vi "Callback Confirm Start.vi"(4 "Variant":variant, 6 "Control Ref":refnum<k7>, 7 "Event Common Data":T1) -> ()   [LabVIEW 2014]
uses:
  support/Message Queue/All Message Queues.ctl
  support/Message Queue/Message Cluster.ctl
  support/Message Queue/Enqueue Message (Single).vi
  support/Message Queue/Message Queue.lvlib
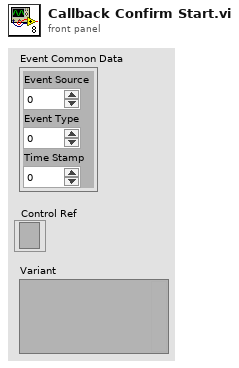
[diagram p1: front panel]
types:
  T1 = cluster{"Event Source":i32, "Event Type":u32, "Time Stamp":u32}
  T2 = typedef "Message Queue.lvlib/All Message Queues.ctl" = cluster{"UI":refnum<queue>, "Engine":refnum<queue>, "Laser":refnum<queue>, "Keyence":refnum<queue>, "Data Processor":refnum<queue>, "Timers":refnum<queue>, "Timer mérés":refnum<queue>, "Timer laser":refnum<queue>, "DAQ":refnum<queue>, "NI Digital":refnum<queue>, "DI data":refnum<queue>, "DO data":refnum<queue>, "Data Processor data":refnum<queue>, "Keyence Data":refnum<queue>, "Ring":refnum<queue>, "NI Analog":refnum<queue>, "AI data":refnum<queue>, "AO data":refnum<queue>, "Analog UI Data":refnum<queue>}
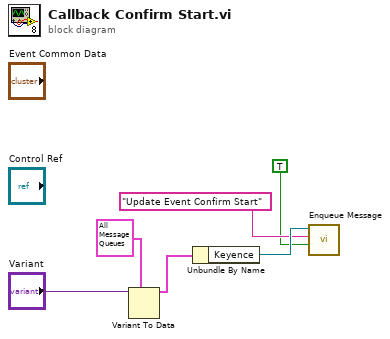
[diagram p0: block diagram]
diagram:
  n1 = Variant To Data(type=T2 {"UI"=refnum, "Engine"=refnum, "Laser"=refnum, "Keyence"=refnum, "Data Processor"=refnum, "Timers"=refnum, "Timer mérés"=refnum, "Timer laser"=refnum, "DAQ"=refnum, "NI Digital"=refnum, "DI data"=refnum, "DO data"=refnum, "Data Processor data"=refnum, "Keyence Data"=refnum, "Ring"=refnum, "NI Analog"=refnum, "AI data"=refnum, "AO data"=refnum, "Analog UI Data"=refnum} ("Message Queues out"), Variant="Variant") -> (data=w5:T2)  [unwired: 1 in, 1 out]
  n2 = Unbundle By Name(w5) -> ("Keyence"=w4:refnum<queue>)
  n3 = call-poly "Enqueue Message.vi"("Message Data"=TRUE, "Message"="Update Event Confirm Start", "Message Queue"=w4) -> ()  [unwired: 7 in, 2 out]
